vi "IOTest.vi"(7 "error in":errorcluster) -> (27 "error out":errorcluster)   [LabVIEW 2016]
uses:
  <vilib>/vision/driver/NI_Vision_Acquisition_Software.lvlib
  <vilib>/vision/NI_Vision_Development_Module.lvlib
panel:
  out "Image Out":T1(plugin-control)
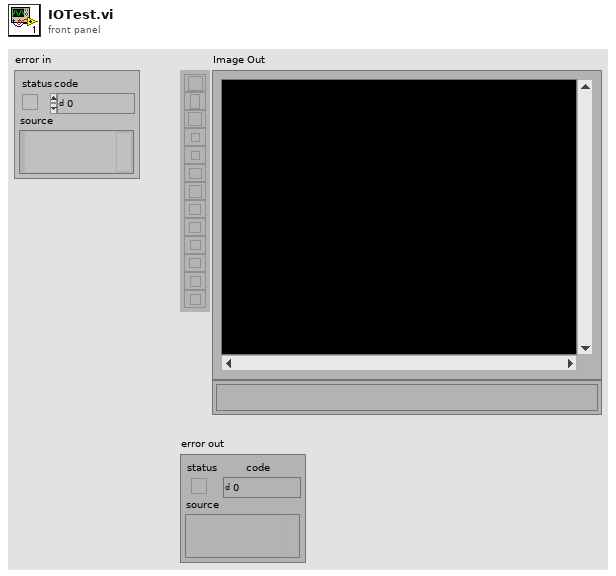
[diagram p1: front panel]
types:
  T1 = typedef "IMAQ Image.ctl" = refnum<image>
  T2 = typedef "IMAQdx.ctl" = refnum<k21>
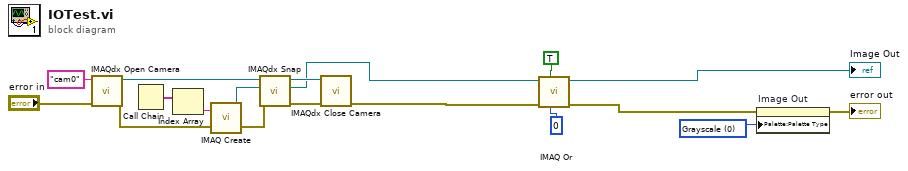
[diagram p0: block diagram]
diagram:
  w1 = u32 0 items=["Grayscale", "Binary", "Gradient", "Rainbow", "Temperature", "User Defined", "Binary 16 Bit", "Gradient 16 Bit", "Rainbow 16 Bit", "Temperature 16 Bit", "User Defined 16 Bit"] ("Palette Type")
  n1 = call <vilib>:"IMAQdx Open Camera.vi"("error in"="error in", "Session In"="cam0" ("Interface Name")) -> ("error out"=w17:errorcluster, "Session Out"=w11:T2)  [unwired: 1 in, 7 out]
  n2 = Call Chain() -> (call chain=w9:string[])
  n3 = Index Array(array=w9) -> (element=w8:string)  [unwired: 1 in]
  n4 = call "IMAQ Create"("Image Name"=w8, "error in (no error)"=w17) -> ("New Image"=w13:T1, "error out"=w12:errorcluster)  [unwired: 2 in, 1 out]
  n5 = call <vilib>:"IMAQdx Snap.vi"("error in"=w12, "Image In"=w13, "Session In"=w11) -> ("error out"=w15:errorcluster, "Image Out"=w5:T1, "Session Out"=w16:T2)  [unwired: 6 out]
  n6 = call <vilib>:"IMAQdx Close Camera.vi"("error in"=w15, "Session In"=w16) -> ("error out"=w14:errorcluster)  [unwired: 9 out]
  n7 = call "IMAQ Or"("Constant"=0, "Or/Nor (Or)"=TRUE, "error in (no error)"=w14, "Image Src A"=w5) -> ("error out"=w4:errorcluster, "Image Dst Out"=→"Image Out":T1)  [unwired: 2 in, 4 out]
  n8 = property on="Image Out" class="ImageControl"(error in=w4, "Palette:Palette Type"=w1) -> (error out=→"error out":errorcluster)  [unwired: 1 in, 1 out]
